vi "PXF4_set_SV.vi"(8 "error in":errorcluster, 10 "SV":dbl, 11 "Modbus Master in":refnum<class "Modbus Master.lvclass">) -> (0 "error out":errorcluster, 3 "Modbus Master out":refnum<class "Modbus Master.lvclass">)   [LabVIEW 2019]
uses:
  <vilib>/NI/Modbus Library/API/Master/Modbus Master.lvclass
panel:
  out "value":dbl
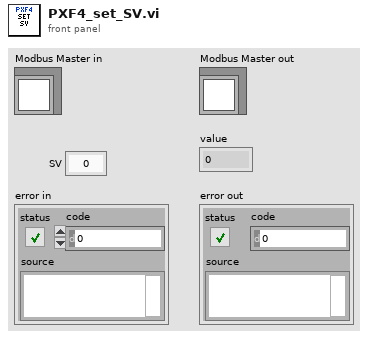
[diagram p1: front panel]
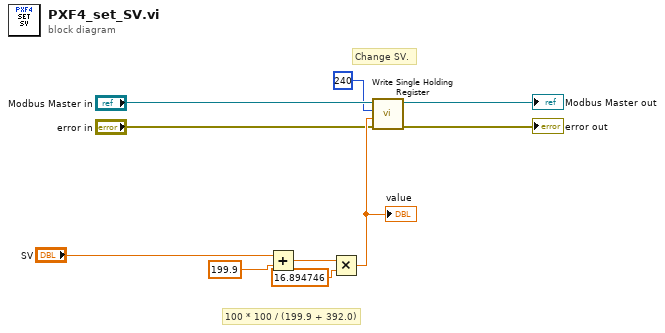
[diagram p0: block diagram]
diagram:
  # "100 * 100 / (199.9 + 392.0)"
  # "Change SV."
  n1 = Add(x="SV", y=199.9 ("value")) -> (x+y=w7:dbl)
  n2 = Multiply(x=w7, y=16.894746) -> (x*y=w9:dbl)
  "value" <- w9
  n3 = call-dynamic "Write Single Holding Register.vi"("error in"="error in", "register to write"=w9, "address"=u16 240, "Modbus master in"="Modbus Master in") -> ("error out"=→"error out":errorcluster, "Modbus master out"=→"Modbus Master out":refnum<class "Modbus Master.lvclass">)  [unwired: 6 in]
